vi "GSP_Manager_Wavelength.vi"() -> ()   [LabVIEW 2015]
uses:
  SystemUtil/Command.ctl
  SystemUtil/ScriptArray.ctl
  SystemUtil/Script.ctl
  wavelength_parameters.ctl
  movetypes.ctl
  SystemUtil/MotorStates.ctl
  SystemUtil/ThreadStates.ctl
  Log/LogItem.ctl
  GSP_Wavelength_Global.vi
  GUI/GSP_GUI_global.vi
panel:
  out "Camera":dbl
  out "Grating":dbl
  out "Array":T1(array[cluster])
  in  "Set":bool
  in  "Load Littrow":bool
  in  "Select Mode:":u16(ring) items=["Custom", "Imaging", "300 All", "600 UV", "600 Blue", "600 Mid", "600 Red", "1200 m0", "1200 m1", "1200 m2", "1200 m3", "1200 m4", "1200 m5", "1200 m6", "1200 m7", "1200 RESOLVE", "400 m1", "400 m2", "930 m1", "930 m2", "930 m3", "930 m4", "930 m5", "930 m6", "400WD", "930TP", "400Fermi", "400Padgett", "400Lewis", "400Crotts", "600BLee", "600RLee", "400WW", "ZZ Ceti Red", "ZZ Ceti Blue"]
  in  "Central wavelength(nm)":dbl
  in  "CS Target":dbl caption="Target" format="%.5f"
  out "CS Angle":dbl caption="Actual" format="%.5f"
  in  "GS Target":dbl caption="Target" format="%.5f"
  out "GS Angle":dbl caption="Actual" format="%.5f"
  out "Last Error":errorcluster
  in  "CommandQ":string
  # "Grating"
  # "Camera"
  # "Littrow Configuration"
  # "Wavelength Angles"
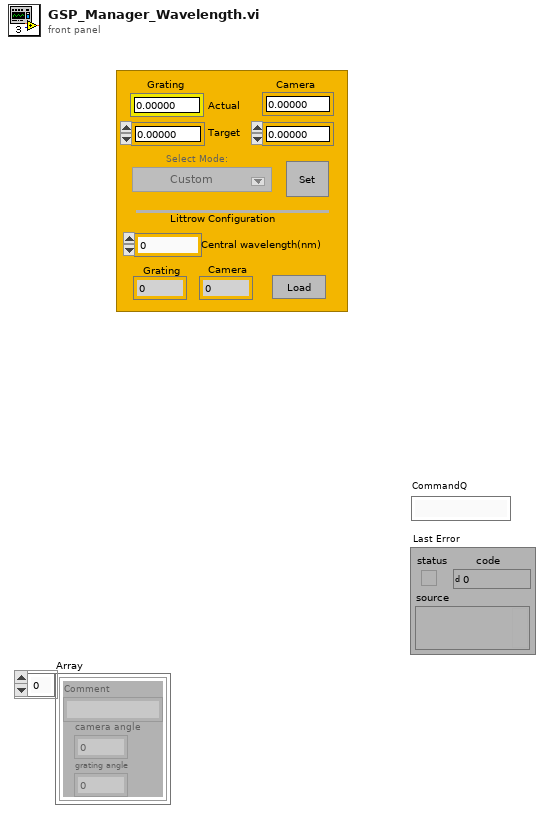
[diagram p1: front panel]
types:
  T1 = cluster{"Comment":string, "camera angle":dbl, "grating angle":dbl}[]
  T2 = typedef "ScriptArray.ctl" = T3[]
  T3 = typedef "Script.ctl" = cluster{"Current Step":i32, "Commands":cluster{"Command":string, "Parameters":string}[]}
  T4 = typedef "Command.ctl" = cluster{"Command":string, "Parameter":string}
  T5 = cluster{"CS - Ext Move Mem Address":i32, "CS - Home Mem Address":i32, "CS - Int Move Mem Address":i32, "GS - Move Mem Address":i32, "GS - Home Mem Address":i32}
  T6 = typedef "wavelength_parameters.ctl" = cluster{"Camera Angle":dbl, "Grating  Angle":dbl, "Move type":T7}
  T7 = typedef "movetypes.ctl" = u16
  T8 = enum16{"POL (0)", "CPL (1)", "HLT (2)", "STP (3)", "RST (4)", "RVN (5)", "RPB (6)", "CLP (8)", "SDL (9)", "RUN (10)", "WRI (11)", "RRG (12)", "SPR (13)", "LPR (14)", "VMI (15)", "SSP (17)", "SSE (18)", "RIS (20)", "RIO (21)", "IMW (25)", "END (128)", "MAV (134)", "MRV (135)", "JRE (137)", "WCL (138)", "WCW (139)", "DLY (140)", "WDL (141)", "GCL (142)", "GOP (143)", "ZTG (144)", "ZTP (145)", "TTP (146)", "CME (147)", "CTC (148)", "TQL (149)", "AHC (150)", "ERL (151)", "OLP (152)", "WRP (154)", "IDT (155)", "LRP (156)", "VMP (159)", "RAV (160)", "RRV (161)", "JMP (162)", "JOI (162)", "CIS (163)", "CKS (164)", "CLC (165)", "KMC (167)", "MCT (168)", "FLC (169)", "EEM (170)", "DDB (171)", "DEM (171)", "PAC (172)", "ADL (173)", "BRT (174)", "MAT (176)", "MRT (177)", "RAT (178)", "RRT (179)", "SSD (180)", "KMR (181)", "KED (182)", "KDD (183)", "DIR (184)", "PRO (185)", "SIF (186)", "EDL (187)", "CIO (188)", "MDS (189)", "MDC (190)", "MDT (191)", "SEE (192)", "ARI (193)", "WBS (194)", "SCF (195)", "RSM (196)", "RLM (197)", "RSN (198)", "RLN (199)", "PCL (201)", "PCI (201)", "PRT (202)", "PRI (202)", "WBE (204)", "SOB (205)", "COB (206)", "ACR (207)", "PLR (208)", "CAI (211)", "LVT (212)", "OVT (213)", "MTT (214)", "CLC (215)", "PIM (216)", "VIM (217)", "TIM (218)", "AHM (219)", "SSL (221)", "TRU (222)", "RSD (223)", "EMT (225)", "DMT (226)", "EMD (227)", "DMD (228)", "HSM (229)", "AHD (230)", "PCM (231)", "PCG (232)", "XRV (233)", "XAV (234)", "XRT (235)", "XAT (236)", "GOC (237)", "JNA (238)", "JOR (239)", "PMC (240)", "PMV (241)", "PMX (242)", "DLC (243)", "SLC (244)", "PCP (245)", "ATR (248)", "PMO (249)", "JAN (250)", "EDH (251)", "DIF (252)", "IMS (253)", "IMQ (254)"}
  T9 = typedef "MotorStates.ctl" = enum16{"Ready", "Moving", "Uninitialized", "Error"}
  T10 = typedef "ThreadStates.ctl" = enum16{"Waiting", "Scripting", "Uninitialized", "Error"}
  T11 = enum16{"Launch", "Log", "Open", "Close", "Shutdown"}
  T12 = typedef "LogItem.ctl" = cluster{"error in (no error)":errorcluster, "Source":string, "Comment ":string}
  T13 = cluster{"Comment":string, "camera angle":dbl, "grating angle":dbl}
  T14 = cluster{"Comment":string, "lines/mm":i32, "modulation":dbl, "thickness (mm)":dbl}
  T15 = cluster{"Mount Az":dbl, "Mount El":dbl, "RA":string, "DEC":string, "Hour Angle":string, "Airmass":dbl, "Focus":dbl, "Rotator Angle":dbl, "Rotator Location":string, "Dome Shutter":string, "Dome Az":dbl, "Date":string, "UT Time":string, "Sidereal Time":string, "Position Angle":dbl, "Seeing":dbl, "OBSRA":string, "OBSDEC":string, "Position ADC":string, "Position ADC 2":string, "Bulb":bool, "Ar":bool, "Cu":bool, "Dome":bool, "Fe":bool, "Hg(Ar)":bool, "Ne":bool, "Quartz":bool, "Dome Percent":dbl, "Quartz Percent":dbl}
  T16 = cluster{"Command":string, "data string":string}[]
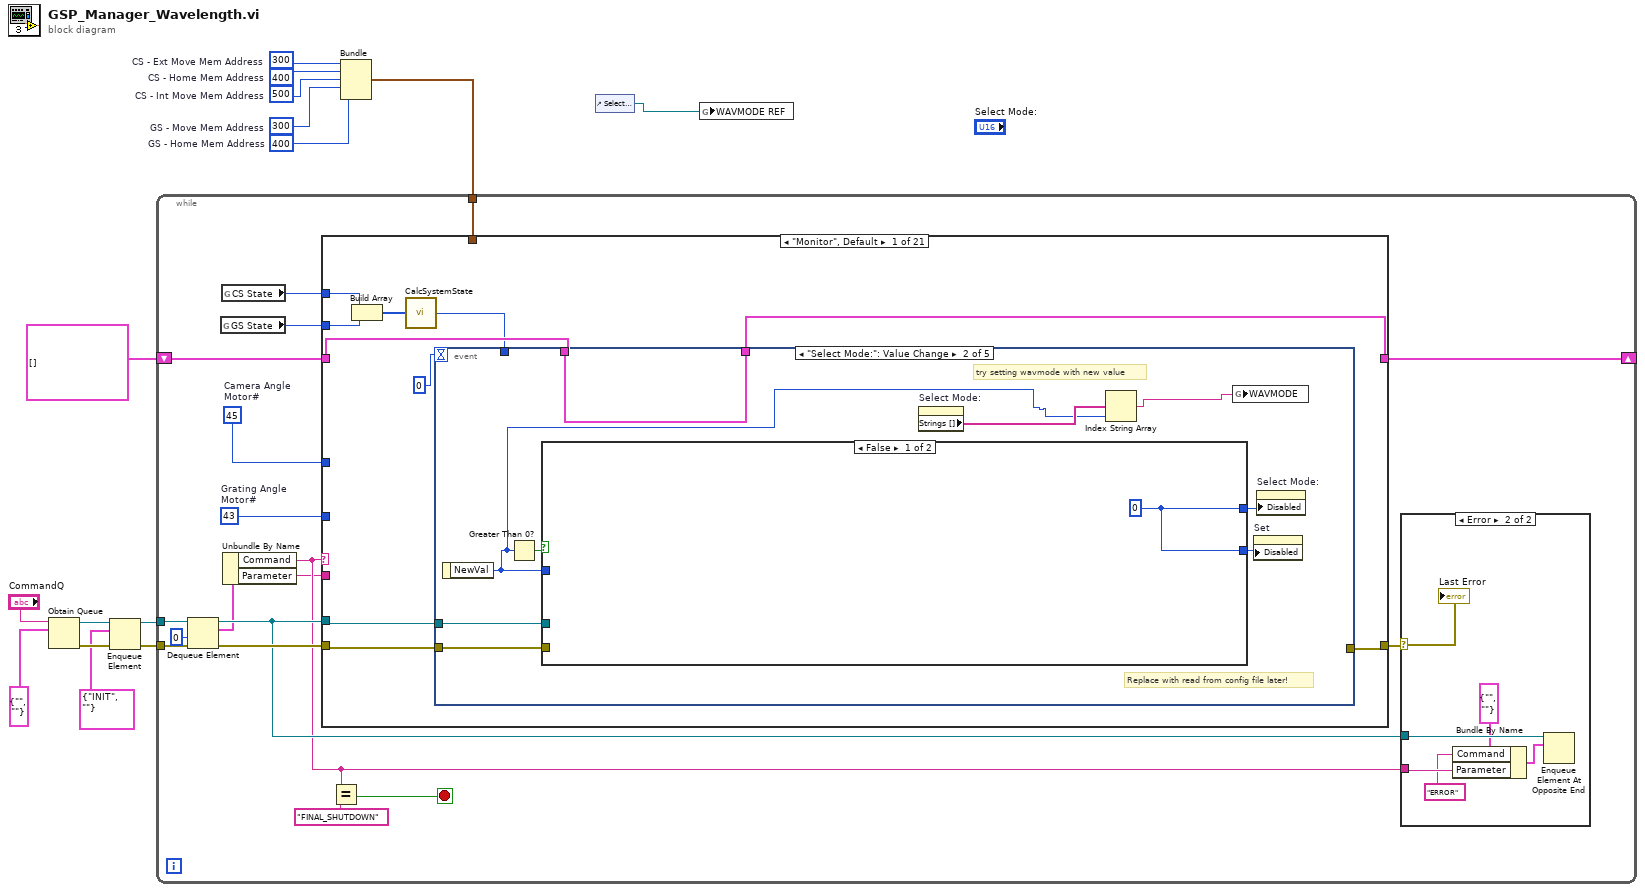
[diagram p0: block diagram]
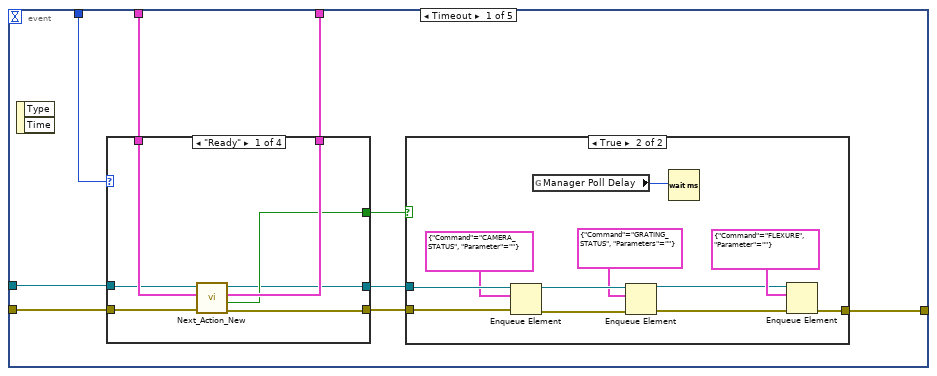
[diagram p3: hidden frame]
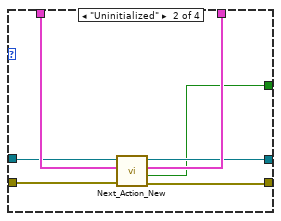
[diagram p5: hidden frame]
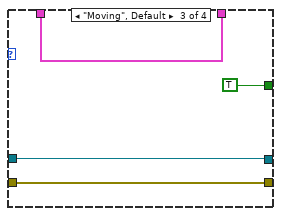
[diagram p6: hidden frame]
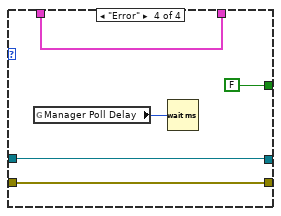
[diagram p7: hidden frame]
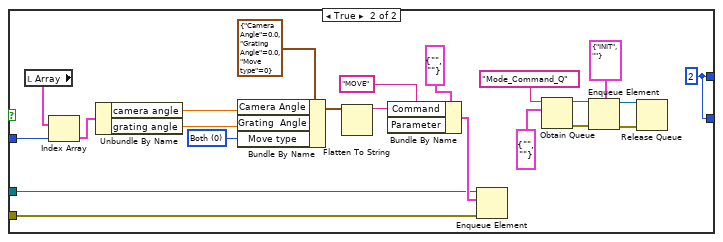
[diagram p8: hidden frame]
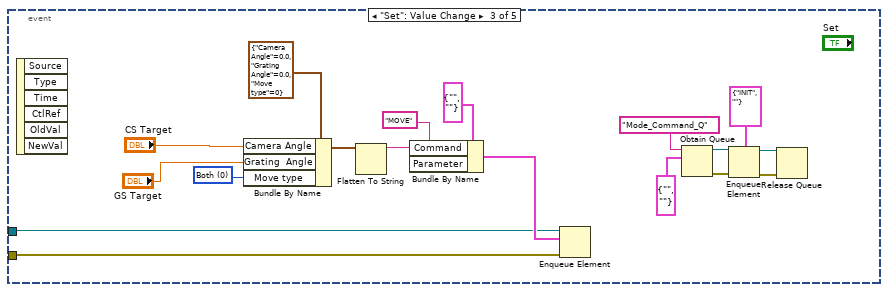
[diagram p9: hidden frame]
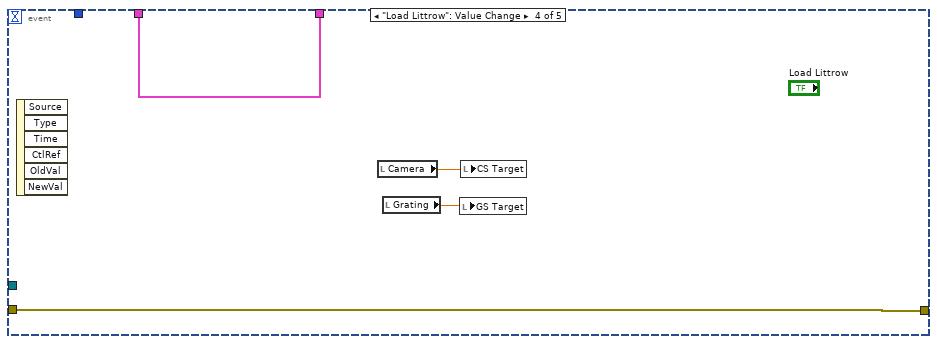
[diagram p10: hidden frame]
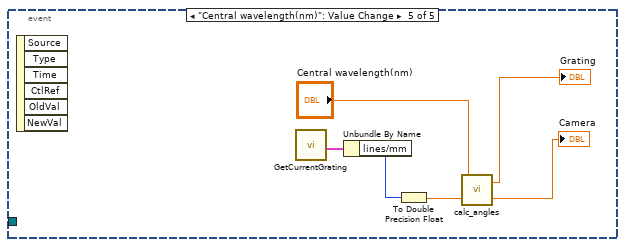
[diagram p11: hidden frame]
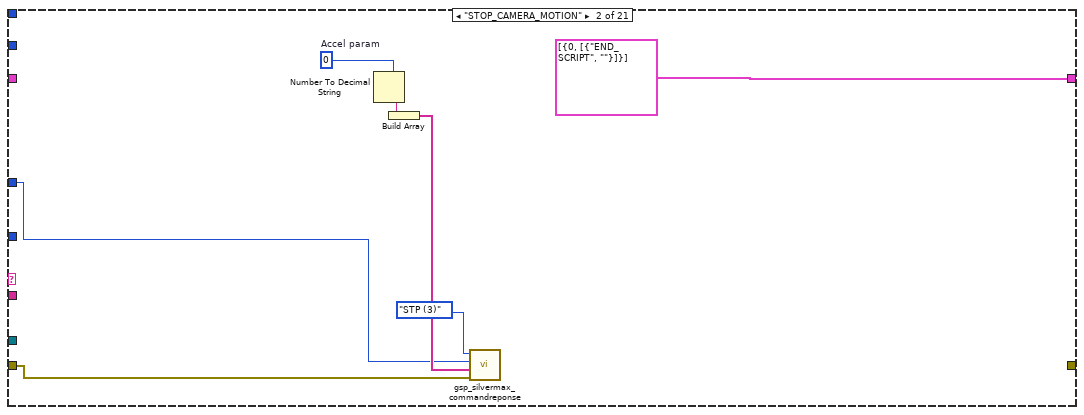
[diagram p12: hidden frame]
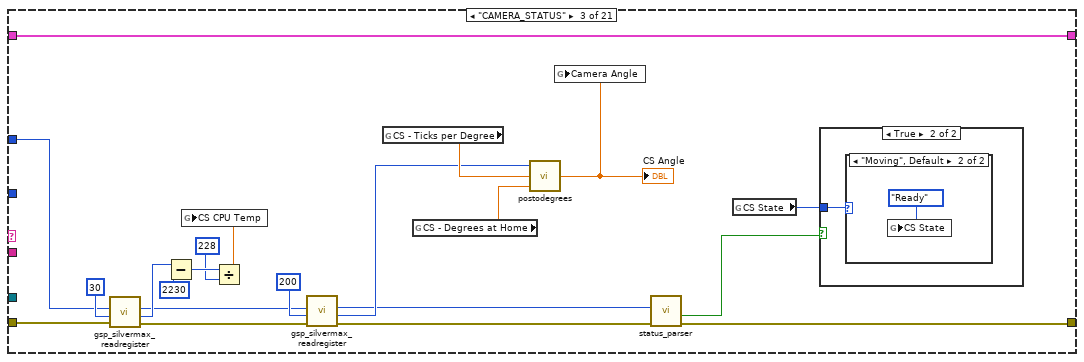
[diagram p13: hidden frame]
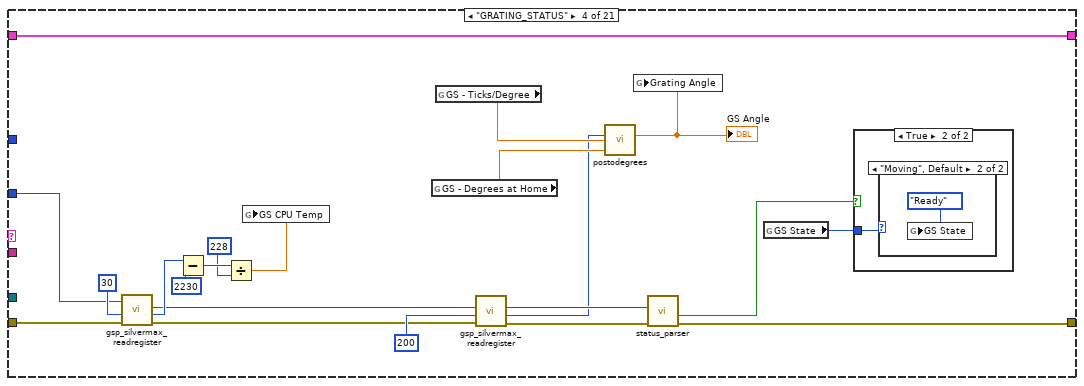
[diagram p16: hidden frame]
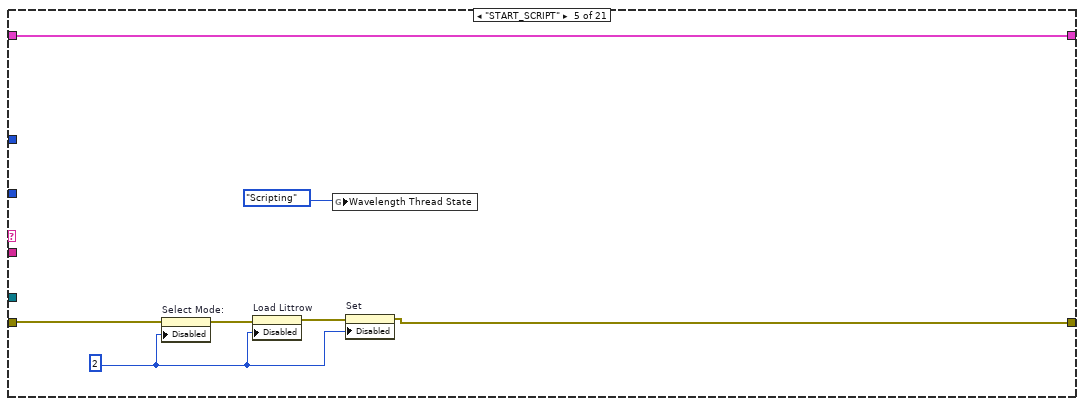
[diagram p19: hidden frame]
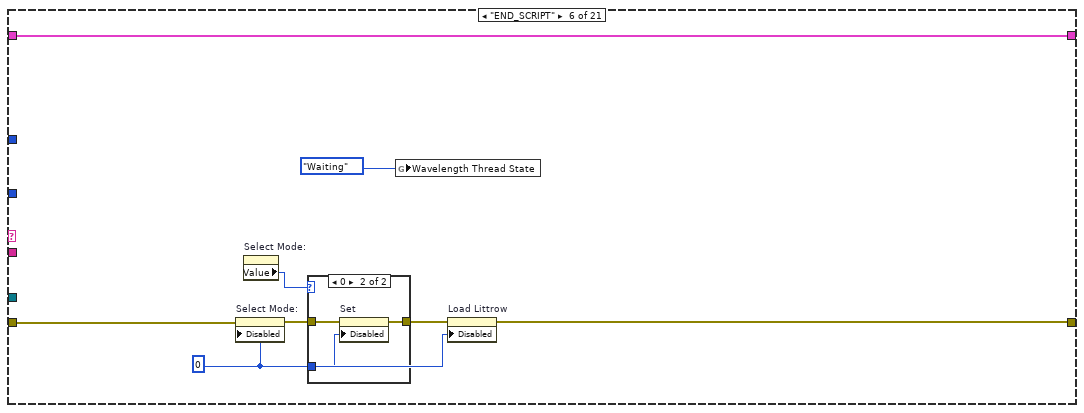
[diagram p20: hidden frame]
diagram:
  w3 = 400  # GS - Home Mem Address
  w6 = 400  # CS - Home Mem Address
  w4 = 300  # GS - Move Mem Address
  w7 = 300  # CS - Ext Move Mem Address
  w5 = 500  # CS - Int Move Mem Address
  n1 = Obtain Queue(name (unnamed)="CommandQ", element data type=T4 {"Command"="", "Parameter"=""} ("Command")) -> (queue out=w13:refnum<queue>, error out=w12:errorcluster)  [unwired: 3 in, 1 out]
  n2 = Enqueue Element(queue=w13, element=T4 {"Command"="INIT", "Parameter"=""}, error in (no error)=w12) -> (queue out=w14:refnum<queue>, error out=w11:errorcluster)  [unwired: 1 in, 1 out]
  n3 = Bundle("CS - Ext Move Mem Address"=w7, "CS - Home Mem Address"=w6, "CS - Int Move Mem Address"=w5, "GS - Move Mem Address"=w4, "GS - Home Mem Address"=w3) -> (w2:T5)  [unwired: 1 in]
  n4 = while {
    tunnel: w14 -> [w33]
    tunnel: w11 -> [w32]
    shift-right: [w25] -> _
    shift-left: T2 [] ("Operations") -> [w27]
    tunnel: w2 -> [w16]
    stop <- w22 stop-if-true
    w21 = u8 43  # Grating Angle Motor#
    w20 = u8 45  # Camera Angle Motor#
    n5 = Dequeue Element(queue=w33, timeout in ms (-1)=0, error in (no error)=w32) -> (queue out=w29:refnum<queue>, element=w24:T4, error out=w31:errorcluster)  [unwired: 1 out]
    n6 = global read "GSP_Wavelength_Global.vi" "GS State"() -> (w17:T9)
    n7 = global read "GSP_Wavelength_Global.vi" "CS State"() -> (w18:T9)
    n8 = Unbundle By Name(w24) -> ("Command"=w23:string, "Parameter"=w19:string)
    n9 = case shown="\"Monitor\", Default" w23 {
      tunnel: w31 -> [w45 w155 w166 w196 w211 w219 w229 w249 w292 w296 w314 _ w362 w384 w406 w429 w469 w515 w522 w523 _]
      tunnel: w29 -> [w46 _ _ _ _ _ _ _ _ _ _ _ _ _ _ _ w471 w514 _ _ w552]
      tunnel: [w49 _ w163 w186 w208 w215 w231 w248 w292 w296 w314 w354 w374 w396 w418 w434 w470 w510 w522 w537 _] -> w30
      tunnel: w27 -> [w48 _ w181 w204 w213 w221 w238 w252 w293 w302 w316 w341 w371 w393 w415 w435 w472 w513 w521 w534 w545]
      tunnel: [w47 T2 [{"Current Step"=0, "Commands"=[{"Command"="END_SCRIPT", "Parameters"=""}]}] ("Operations") w181 w204 w213 w221 w238 w250 w293 w301 w315 w341 w371 w393 w415 w435 w468 w513 w520 w534 w544] -> w25
      tunnel: w19 -> [_ _ _ _ _ _ _ w251 _ _ _ w348 w369 w391 w414 w452 _ _ _ _ _]
      tunnel: w21 -> [_ _ _ w197 _ _ _ _ _ _ _ _ _ _ w409 w438 _ _ _ w527 _]
      tunnel: w20 -> [_ w156 w167 _ _ _ _ _ _ _ _ w344 w370 w392 _ w449 _ _ _ w528 _]
      tunnel: w18 -> [w44 _ _ _ _ _ _ w246 _ _ w311 _ _ _ _ _ _ _ _ _ _]
      tunnel: w17 -> [w43 _ _ _ _ _ _ w245 _ _ w310 _ _ _ _ _ _ _ _ _ _]
      tunnel: w16 -> [_ _ _ _ _ _ _ _ _ _ _ w343 w364 w386 w408 w448 _ _ _ w526 _]
      frame "Monitor", Default {
        n10 = Build Array(w44, w43) -> (w42:T9[])
        n11 = call "CalcSystemState.vi"("Motor States"=w42) -> ("system state"=w41:T9)
        n12 = event shown="[1] \"Select Mode:\": Value Change" {
          selector: _ -> [_ _ _ _ _]
          dyn-events: _ -> [_ _ _ _ _]
          timeout: 0 -> [_ _ _ _ _]
          tunnel: [w55 _ _ w147 _] -> w49
          tunnel: w48 -> [w54 w100 _ w146 _]
          tunnel: [w53 w100 _ w146 _] -> w47
          tunnel: w46 -> [w52 w102 w137 _ _]
          tunnel: w45 -> [w51 w101 w136 w147 _]
          tunnel: w41 -> [w50 _ _ _ _]
          event Timeout {
            n13 = event-data() -> ()  [unwired: 1 in, 2 out]
            n14 = case shown="\"Ready\"" w50 {
              tunnel: w52 -> [w73 w80 w87 w90]
              tunnel: w51 -> [w77 w84 w86 w92]
              tunnel: [w75 w82 w86 w92] -> w58
              tunnel: w54 -> [w76 w83 w88 w93]
              tunnel: [w74 w81 w88 w93] -> w53
              tunnel: [w72 w78 TRUE FALSE] -> w57
              tunnel: [w71 w79 w87 w90] -> w56
              frame "Ready" {
                n15 = call "Next_Action_New.vi"("error in (no error)"=w77, "Operations"=w76, "queue in"=w73) -> ("error out"=w75:errorcluster, "No command?"=w72:bool, "Operations Out"=w74:T2, "queue out"=w71:refnum<queue>)  [unwired: 1 in]
              }
              frame "Uninitialized" {
                n16 = call "Next_Action_New.vi"("error in (no error)"=w84, "Operations"=w83, "queue in"=w80) -> ("error out"=w82:errorcluster, "No command?"=w78:bool, "Operations Out"=w81:T2, "queue out"=w79:refnum<queue>)  [unwired: 1 in]
              }
              frame "Moving", Default {
              }
              frame "Error" {
                n17 = global read "GSP_GUI_global.vi" "Manager Poll Delay"() -> (w91:u32)
                n18 = Wait (ms)(milliseconds to wait=w91) -> ()  [unwired: 1 out]
              }
            }
            n19 = case shown="True" w57 {
              tunnel: w58 -> [w59 w70]
              tunnel: w56 -> [_ w69]
              tunnel: [w59 w60] -> w55
              frame False {
              }
              frame True {
                n20 = Enqueue Element(queue=w69, element=T4 {"Command"="CAMERA_STATUS", "Parameter"=""}, error in (no error)=w70) -> (queue out=w67:refnum<queue>, error out=w66:errorcluster)  [unwired: 1 in, 1 out]
                n21 = global read "GSP_GUI_global.vi" "Manager Poll Delay"() -> (w68:u32)
                n22 = Enqueue Element(queue=w67, element=cluster{"Command":string, "Parameters":string} {"Command"="GRATING_STATUS", "Parameters"=""} ("Default Command"), error in (no error)=w66) -> (queue out=w62:refnum<queue>, error out=w61:errorcluster)  [unwired: 1 in, 1 out]
                n23 = Wait (ms)(milliseconds to wait=w68) -> ()  [unwired: 1 out]
                n24 = Enqueue Element(queue=w62, element=T4 {"Command"="FLEXURE", "Parameter"=""}, error in (no error)=w61) -> (error out=w60:errorcluster)  [unwired: 1 in, 2 out]
              }
            }
          }
          event "Select Mode:": Value Change {
            # "try setting wavmode with new value"
            # "Replace with read from config file later!"
            n25 = event-data() -> ("NewVal"=w94:u16)  [unwired: 1 in]
            n26 = Greater Than 0?(x=w94) -> (x > 0?=w99:bool)
            n27 = case shown="False" w99 {
              tunnel: w94 -> [_ w115]
              tunnel: w102 -> [_ w118]
              tunnel: w101 -> [_ w117]
              tunnel: [w103 w116] -> w98
              tunnel: [w103 w116] -> w97
              frame False {
                w103 = u8 0 ("Disabled")
              }
              frame True {
                w116 = u8 2 ("Disabled")
                w119 = T7 0 items=["Both", "Grating Only", "Camera Only"] ("Move type")
                n28 = local read "Array"() -> (w114:T1)
                n29 = Index Array(array=w114, index=w115) -> (element=w113:T13)
                n30 = Unbundle By Name(w113) -> ("camera angle"=w112:dbl, "grating angle"=w111:dbl)
                n31 = Bundle By Name(cluster=T6 {"Camera Angle"=0.0, "Grating  Angle"=0.0, "Move type"=0} ("Wavelength Parameters"), "Camera Angle"=w112, "Grating  Angle"=w111, "Move type"=w119) -> (w120:T6)
                n32 = Flatten To String(anything=w120) -> (data string=w123:string)  [unwired: 3 in, 2 out]
                n33 = Bundle By Name(cluster=T4 {"Command"="", "Parameter"=""} ("element"), "Command"="MOVE", "Parameter"=w123) -> (w124:T4)
                n34 = Enqueue Element(queue=w118, element=w124, error in (no error)=w117) -> ()  [unwired: 1 in, 3 out]
                n35 = Obtain Queue(name (unnamed)="Mode_Command_Q", element data type=T4 {"Command"="", "Parameter"=""} ("element")) -> (queue out=w110:refnum<queue>, error out=w109:errorcluster)  [unwired: 3 in, 1 out]
                n36 = Enqueue Element(queue=w110, element=T4 {"Command"="INIT", "Parameter"=""}, error in (no error)=w109) -> (queue out=w105:refnum<queue>, error out=w104:errorcluster)  [unwired: 1 in, 1 out]
                n37 = Release Queue(queue=w105, error in (no error)=w104) -> ()  [unwired: 1 in, 3 out]
              }
            }
            n38 = property on="Select Mode:" class="Ring (strict)"() -> ("Strings []"=w96:string[])  [unwired: 2 in, 2 out]
            n39 = Index String Array(1:w94, 2:w96) -> (0:w95:string)  [unwired: 1 in]
            n40 = global write "GSP_Wavelength_Global.vi" "WAVMODE"(w95) -> ()
            n41 = property on="Set" class="Bool"("Disabled"=w97) -> ()  [unwired: 2 in, 2 out]
            n42 = property on="Select Mode:" class="Ring (strict)"("Disabled"=w98) -> ()  [unwired: 2 in, 2 out]
          }
          event "Set": Value Change {
            w138 = T7 0 items=["Both", "Grating Only", "Camera Only"] ("Move type")
            n43 = event-data() -> ()  [unwired: 1 in, 6 out]
            n44 = Bundle By Name(cluster=T6 {"Camera Angle"=0.0, "Grating  Angle"=0.0, "Move type"=0} ("Wavelength Parameters"), "Camera Angle"="CS Target", "Grating  Angle"="GS Target", "Move type"=w138) -> (w139:T6)
            n45 = Flatten To String(anything=w139) -> (data string=w141:string)  [unwired: 3 in, 2 out]
            n46 = Bundle By Name(cluster=T4 {"Command"="", "Parameter"=""} ("element"), "Command"="MOVE", "Parameter"=w141) -> (w142:T4)
            n47 = Enqueue Element(queue=w137, element=w142, error in (no error)=w136) -> ()  [unwired: 1 in, 3 out]
            n48 = Obtain Queue(name (unnamed)="Mode_Command_Q", element data type=T4 {"Command"="", "Parameter"=""} ("element")) -> (queue out=w132:refnum<queue>, error out=w131:errorcluster)  [unwired: 3 in, 1 out]
            n49 = Enqueue Element(queue=w132, element=T4 {"Command"="INIT", "Parameter"=""}, error in (no error)=w131) -> (queue out=w127:refnum<queue>, error out=w126:errorcluster)  [unwired: 1 in, 1 out]
            n50 = Release Queue(queue=w127, error in (no error)=w126) -> ()  [unwired: 1 in, 3 out]
          }
          event "Load Littrow": Value Change {
            n51 = event-data() -> ()  [unwired: 1 in, 6 out]
            n52 = local read "Camera"() -> (w145:dbl)
            n53 = local read "Grating"() -> (w144:dbl)
            n54 = local write "GS Target"(w144) -> ()
            n55 = local write "CS Target"(w145) -> ()
          }
          event "Central wavelength(nm)": Value Change {
            n56 = event-data() -> ()  [unwired: 1 in, 6 out]
            n57 = call "GetCurrentGrating.vi"() -> ("Current Grating"=w153:T14)
            n58 = Unbundle By Name(w153) -> ("lines/mm"=w151:i32)
            n59 = To Double Precision Float(number=w151) -> (double precision float=w152:dbl)
            n60 = call "calc_angles.vi"("lines/mm"=w152, "Central Wavlength (nm)"="Central wavelength(nm)") -> ("camera angle"=→"Camera":dbl, "grating angle"=→"Grating":dbl)
          }
        }
      }
      frame "STOP_CAMERA_MOTION" {
        w159 = u8 0  # Accel param
        n61 = Number To Decimal String(number=w159) -> (decimal integer string=w160:string)  [unwired: 1 in]
        n62 = Build Array(w160) -> (w157:string[])
        n63 = call "gsp_silvermax_commandreponse.vi"("error in (no error)"=w155, "Parameters (none)"=w157, "Motor #"=w156, "Command"=T8."STP (3)") -> ()  [unwired: 4 out]
      }
      frame "CAMERA_STATUS" {
        n64 = call "gsp_silvermax_readregister.vi"("error in (no error)"=w166, "Register# (0)"=u8 30, "Motor #"=w167) -> ("error out"=w165:errorcluster, "Register Value"=w172:i32, "Motor # dup"=w164:u8)  [unwired: 2 in, 2 out]
        n65 = Subtract(x=w172, y=2230) -> (x-y=w171:i32)
        n66 = Divide(x=w171, y=228) -> (x/y=w169:dbl)
        n67 = global write "GSP_Wavelength_Global.vi" "CS CPU Temp"(w169) -> ()
        n68 = call "gsp_silvermax_readregister.vi"("error in (no error)"=w165, "Register# (0)"=u8 200, "Motor #"=w164) -> ("error out"=w179:errorcluster, "Register Value"=w176:i32, "Motor # dup"=w174:u8)  [unwired: 2 in, 2 out]
        n69 = global read "GSP_Wavelength_Global.vi" "CS - Ticks per Degree"() -> (w178:dbl)
        n70 = global read "GSP_Wavelength_Global.vi" "CS - Degrees at Home"() -> (w177:dbl)
        n71 = call "postodegrees.vi"("Degrees @ Home (15.00)"=w177, "Ticks per degree (28571.43)"=w178, "Ext Position"=w176) -> ("Degrees"=w161:dbl)  [unwired: 2 in]
        "CS Angle" <- w161
        n72 = global write "GSP_Wavelength_Global.vi" "Camera Angle"(w161) -> ()
        n73 = call "status_parser.vi"("error in (no error)"=w179, "Motor #"=w174) -> ("error out"=w163:errorcluster, "Program Complete?"=w180:bool)  [unwired: 3 in, 1 out]
        n74 = global read "GSP_Wavelength_Global.vi" "CS State"() -> (w162:T9)
        n75 = case shown="True" w180 {
          tunnel: w162 -> [_ w182]
          frame False {
          }
          frame True {
            n76 = case shown="\"Moving\", Default" w182 {
              frame "Uninitialized" {
              }
              frame "Moving", Default {
                n77 = global write "GSP_Wavelength_Global.vi" "CS State"(MotorStates."Ready" ("Mode")) -> ()
              }
            }
          }
        }
      }
      frame "GRATING_STATUS" {
        n78 = call "gsp_silvermax_readregister.vi"("error in (no error)"=w196, "Register# (0)"=u8 30, "Motor #"=w197) -> ("error out"=w188:errorcluster, "Register Value"=w202:i32, "Motor # dup"=w187:u8)  [unwired: 2 in, 2 out]
        n79 = Subtract(x=w202, y=2230) -> (x-y=w201:i32)
        n80 = Divide(x=w201, y=228) -> (x/y=w199:dbl)
        n81 = global write "GSP_Wavelength_Global.vi" "GS CPU Temp"(w199) -> ()
        n82 = global read "GSP_Wavelength_Global.vi" "GS - Degrees at Home"() -> (w191:dbl)
        n83 = global read "GSP_Wavelength_Global.vi" "GS - Ticks/Degree"() -> (w192:dbl)
        n84 = call "gsp_silvermax_readregister.vi"("error in (no error)"=w188, "Register# (0)"=u8 200, "Motor #"=w187) -> ("error out"=w195:errorcluster, "Register Value"=w190:i32, "Motor # dup"=w194:u8)  [unwired: 2 in, 2 out]
        n85 = call "postodegrees.vi"("Degrees @ Home (15.00)"=w191, "Ticks per degree (28571.43)"=w192, "Ext Position"=w190) -> ("Degrees"=w184:dbl)  [unwired: 2 in]
        "GS Angle" <- w184
        n86 = global write "GSP_Wavelength_Global.vi" "Grating Angle"(w184) -> ()
        n87 = call "status_parser.vi"("error in (no error)"=w195, "Motor #"=w194) -> ("error out"=w186:errorcluster, "Program Complete?"=w193:bool)  [unwired: 3 in, 1 out]
        n88 = global read "GSP_Wavelength_Global.vi" "GS State"() -> (w185:T9)
        n89 = case shown="True" w193 {
          tunnel: w185 -> [_ w205]
          frame False {
          }
          frame True {
            n90 = case shown="\"Moving\", Default" w205 {
              frame "Uninitialized" {
              }
              frame "Moving", Default {
                n91 = global write "GSP_Wavelength_Global.vi" "GS State"(MotorStates."Ready" ("Grating Mode")) -> ()
              }
            }
          }
        }
      }
      frame "START_SCRIPT" {
        w207 = u8 2 ("Disabled")
        n92 = property on="Select Mode:" class="Ring (strict)"(error in=w211, "Disabled"=w207) -> (error out=w210:errorcluster)  [unwired: 1 in, 1 out]
        n93 = property on="Load Littrow" class="Bool"(error in=w210, "Disabled"=w207) -> (error out=w209:errorcluster)  [unwired: 1 in, 1 out]
        n94 = global write "GSP_Wavelength_Global.vi" "Wavelength Thread State"(ThreadStates."Scripting" ("Thread state")) -> ()
        n95 = property on="Set" class="Bool"(error in=w209, "Disabled"=w207) -> (error out=w208:errorcluster)  [unwired: 1 in, 1 out]
      }
      frame "END_SCRIPT" {
        w218 = u8 0 ("Disabled")
        n96 = property on="Select Mode:" class="Ring (strict)"(error in=w219, "Disabled"=w218) -> (error out=w217:errorcluster)  [unwired: 1 in, 1 out]
        n97 = property on="Select Mode:" class="Ring (strict)"() -> ("Value"=w214:u16)  [unwired: 2 in, 2 out]
        n98 = case shown="0" w214 {
          tunnel: w218 -> [_ w225]
          tunnel: w217 -> [w222 w224]
          tunnel: [w222 w223] -> w216
          frame 1, Default {
          }
          frame 0 {
            n99 = property on="Set" class="Bool"(error in=w224, "Disabled"=w225) -> (error out=w223:errorcluster)  [unwired: 1 in, 1 out]
          }
        }
        n100 = global write "GSP_Wavelength_Global.vi" "Wavelength Thread State"(ThreadStates."Waiting" ("Thread state")) -> ()
        n101 = property on="Load Littrow" class="Bool"(error in=w216, "Disabled"=w218) -> (error out=w215:errorcluster)  [unwired: 1 in, 1 out]
      }
      frame "INIT" {
        w232 = u8 2 ("Disabled")
        w237 = MotorStates."Uninitialized" ("Camera Mode")
        n102 = global read "GSP_GUI_global.vi" "Standard Observing Mode Names"() -> (w227:string[])
        n103 = global read "GSP_GUI_global.vi" "Standard Observing Modes File"() -> (w230:path)
        n104 = for {
          tunnel: w227 -> [w243] mode=indexing
          tunnel: w230 -> [w244]
          tunnel: w229 -> [w242]
          tunnel: [w241] -> w228
          tunnel: [w240] -> w226 mode=indexing
          n105 = call "get_std_observing_modes.vi"("error in (no error)"=w242, "mode name"=w243, "configuration file path"=w244) -> ("error out"=w241:errorcluster, "Standard Mode Info"=w240:T13)  [unwired: 3 in]
        }
        "Array" <- w226
        n106 = property on="Select Mode:" class="Ring (strict)"(error in=w228, "Disabled"=w232) -> (error out=w234:errorcluster)  [unwired: 1 in, 1 out]
        n107 = property on="Select Mode:" class="Ring (strict)"("Strings []"=w227) -> ()  [unwired: 2 in, 2 out]
        n108 = property on="Set" class="Bool"(error in=w234, "Disabled"=w232) -> (error out=w233:errorcluster)  [unwired: 1 in, 1 out]
        n109 = property on="Load Littrow" class="Bool"(error in=w233, "Disabled"=w232) -> (error out=w231:errorcluster)  [unwired: 1 in, 1 out]
        n110 = global write "GSP_Wavelength_Global.vi" "Flexure Active"(FALSE ("Flexure Active")) -> ()
        n111 = global write "GSP_Wavelength_Global.vi" "WL Online"(TRUE ("CS Online")) -> ()
        n112 = global write "GSP_Wavelength_Global.vi" "Wavelength Thread State"(ThreadStates."Uninitialized" ("Thread state")) -> ()
        n113 = global write "GSP_Wavelength_Global.vi" "CS State"(w237) -> ()
        n114 = global write "GSP_Wavelength_Global.vi" "GS State"(w237) -> ()
      }
      frame "MOVE" {
        n115 = call "Slit_allow_move.vi"("Translation Mode"=w246, "Rotation Mode"=w245) -> ("Allow Move?"=w247:bool)
        n116 = case shown="True" w247 {
          tunnel: w252 -> [w269 w284]
          tunnel: w251 -> [w267 _]
          tunnel: [w268 w284] -> w250
          tunnel: w249 -> [w256 w289]
          tunnel: [w257 w288] -> w248
          frame True {
            n117 = Unflatten From String(type=T6 {"Camera Angle"=0.0, "Grating  Angle"=0.0, "Move type"=0} ("Wavelength Parameters"), binary string=w267) -> (value=w265:T6)  [unwired: 3 in, 2 out]
            n118 = global read "GSP_Wavelength_Global.vi" "Grating Angle"() -> (w255:dbl)
            n119 = global read "GSP_Wavelength_Global.vi" "Camera Angle"() -> (w254:dbl)
            n120 = Unbundle By Name(w265) -> ("Move type"=w253:T7, "Grating  Angle"=w259:dbl, "Camera Angle"=w258:dbl)
            n121 = call "GSP_Wavelength_GenerateScript.vi"("Current Grating"=w255, "Current Camera"=w254, "Target Grating"=w259, "Target Camera"=w258, "Move type"=w253) -> ("Script"=w263:cluster{string, string}[], "AllowMove?"=w264:bool)
            n122 = Build Array (concatenate)(cluster{string, string} {"START_SCRIPT", ""}, w263, cluster{string, string} {"END_SCRIPT", ""}) -> (w261:cluster{string, string}[])
            n123 = case shown="True" w264 {
              tunnel: w269 -> [w276 w281]
              tunnel: [w276 w279] -> w268
              tunnel: w261 -> [_ w278]
              tunnel: w259 -> [_ _]
              tunnel: w258 -> [_ _]
              tunnel: [w271 w277] -> w257
              tunnel: w256 -> [w272 w277]
              frame False {
                w274 = T12 {"error in (no error)"={"status"=FALSE, "code"=0, "source"=""}, "Source"="", "Comment "=""} ("Log")
                n124 = Bundle By Name(cluster=w274, "Comment"="Move request out of bounds", "Source"="Wavlength Manager") -> ()  [unwired: 1 out]
                n125 = call "GSP_Logger_Handler.vi"("error in (no error)"=w272, "Log"=w274, "Actions"=T11."Log") -> ("error out"=w271:errorcluster)  [unwired: 4 in]
              }
              frame True {
                n126 = call "Build_Script.vi"("Commands"=w278) -> ("script out"=w280:T3)  [unwired: 4 in]
                n127 = Insert Into Array(array=w281, new element=w280) -> (w279:T2)  [unwired: 1 in]
              }
            }
          }
          frame False {
            n128 = Bundle By Name(cluster=T12 {"error in (no error)"={"status"=FALSE, "code"=0, "source"=""}, "Source"="", "Comment "=""} ("Log"), "Source"="Wavelength Manager", "Comment"="Cannot perform move") -> (w285:T12)
            n129 = call "GSP_Logger_Handler.vi"("error in (no error)"=w289, "Log"=w285, "Actions"=T11."Log") -> ("error out"=w288:errorcluster)  [unwired: 4 in]
          }
        }
      }
      frame "FLEXURE_ON" {
        n130 = global read "GSP_Wavelength_Global.vi" "Camera Target"() -> (w290:dbl)
        n131 = global write "GSP_Wavelength_Global.vi" "Flexure Active"(TRUE) -> ()
        n132 = global write "GSP_Wavelength_Global.vi" "Camera Flex Target"(w290) -> ()
      }
      frame "FLEXURE_OFF" {
        n133 = global read "GSP_Wavelength_Global.vi" "Camera Target"() -> (w295:dbl)
        n134 = Flatten To String(anything=w295) -> (data string=w294:string)  [unwired: 3 in, 2 out]
        n135 = global write "GSP_Wavelength_Global.vi" "Flexure Active"(FALSE) -> ()
        n136 = Bundle By Name(cluster=T4 {"Command"="", "Parameter"=""} ("element"), "Command"="CAMERA_EXT_MOVE_START", "Parameter"=w294) -> (w297:T4)
        n137 = Build Array(cluster{string, string} {"START_SCRIPT", ""}, w297, cluster{string, string} {"END_SCRIPT", ""}) -> (w299:T4[])
        n138 = call "Build_Script.vi"("Commands"=w299) -> ("script out"=w303:T3)  [unwired: 4 in]
        n139 = Insert Into Array(array=w302, new element=w303) -> (w301:T2)  [unwired: 1 in]
      }
      frame "FLEXURE" {
        n140 = Build Array(w311, w310) -> (w312:T9[])
        n141 = global read "GSP_Wavelength_Global.vi" "Flexure Active"() -> (w313:bool)
        n142 = call "CalcSystemState.vi"("Motor States"=w312) -> ("system state"=w309:T9)
        n143 = Equal?(x=w309, y=MotorStates."Ready") -> (x = y?=w307:bool)
        n144 = And(x=w307, y=w313) -> (x .and. y?=w317:bool)
        n145 = case shown="True" w317 {
          tunnel: w316 -> [w318 w328]
          tunnel: [w318 w327] -> w315
          frame False {
          }
          frame True {
            n146 = call "GetTCSInfo.vi"() -> ("TCSInfo"=w320:T15)
            n147 = global read "GSP_Wavelength_Global.vi" "Camera Flex Target"() -> (w322:dbl)
            n148 = global read "GSP_Wavelength_Global.vi" "Camera Target"() -> (w329:dbl)
            n149 = global read "GSP_Wavelength_Global.vi" "B1"() -> (w330:dbl)
            n150 = Unbundle By Name(w320) -> ("Rotator Angle"=w319:dbl)
            n151 = call "CalcCameraFlex.vi"("Camera Target"=w329, "B1"=w330, "Rotator Position"=w319) -> ("Camera Flex Target"=w325:dbl)  [unwired: 1 out]
            n152 = global read "GSP_Wavelength_Global.vi" "Flex_Max"() -> (w326:dbl)
            n153 = Subtract(x=w325, y=w322) -> (x-y=w324:dbl)
            n154 = Absolute Value(x=w324) -> (abs(x)=w323:dbl)
            n155 = Greater?(x=w323, y=w326) -> (0:w321:bool)
            n156 = case shown="True" w321 {
              tunnel: w328 -> [w331 w333]
              tunnel: w325 -> [_ w334]
              tunnel: [w331 w335] -> w327
              frame False {
              }
              frame True {
                n157 = Flatten To String(anything=w334) -> (data string=w336:string)  [unwired: 3 in, 2 out]
                n158 = Bundle("Command"="CAMERA_FLEX_MOVE_START", "data string"=w336) -> (w337:cluster{"Command":string, "data string":string})  [unwired: 1 in]
                n159 = Build Array(w337) -> (w332:T16)
                n160 = call "Build_Script.vi"("Commands"=w332) -> ("script out"=w338:T3)  [unwired: 4 in]
                n161 = Insert Into Array(array=w333, new element=w338) -> (w335:T2)  [unwired: 1 in]
              }
            }
          }
        }
      }
      frame "CAMERA_INT_MOVE_START" {
        w347 = 0.0  # Degrees
        n162 = Unflatten From String(type=w347, binary string=w348) -> (value=w340:dbl)  [unwired: 3 in, 2 out]
        n163 = Unbundle By Name(w343) -> ("CS - Int Move Mem Address"=w342:i32)
        n164 = global write "GSP_Wavelength_Global.vi" "Camera Target"(w340) -> ()
        n165 = local write "CS Target"(w340) -> ()
        n166 = global read "GSP_Wavelength_Global.vi" "CS - Degrees at Home"() -> (w346:dbl)
        n167 = call "degreestopos.vi"("Degrees @ Home (15.00)"=w346, "Ticks per degree (28571.43)"=1960.0, "Degrees"=w340) -> ("Position"=w351:i32)  [unwired: 2 in]
        n168 = Number To Decimal String(number=w342) -> (decimal integer string=w353:string)  [unwired: 1 in]
        n169 = call "gsp_silvermax_writeregister.vi"("Register Value"=w351, "Motor #"=w344, "Register# (0)"=u8 25) -> ("error out"=w356:errorcluster, "Motor # dup"=w355:u8)  [unwired: 3 in]
        n170 = Build Array(w353) -> (w352:string[])
        n171 = call "gsp_silvermax_commandreponse.vi"("error in (no error)"=w356, "Parameters (none)"=w352, "Motor #"=w355, "Command"=T8."LRP (156)") -> ("error out"=w349:errorcluster)  [unwired: 3 out]
        n172 = case shown="No Error" w349 {
          selector: w349 -> [w359 w360]
          tunnel: [w359 w360] -> w354
          frame No Error {
            n173 = global write "GSP_Wavelength_Global.vi" "CS State"(MotorStates."Moving" ("Mode")) -> ()
          }
          frame Error {
          }
        }
      }
      frame "CAMERA_EXT_MOVE_START" {
        w368 = 0.0  # Degrees
        n174 = Unflatten From String(type=w368, binary string=w369) -> (value=w361:dbl)  [unwired: 3 in, 2 out]
        n175 = global write "GSP_Wavelength_Global.vi" "Camera Target"(w361) -> ()
        n176 = Unbundle By Name(w364) -> ("CS - Ext Move Mem Address"=w363:i32)
        n177 = local write "CS Target"(w361) -> ()
        n178 = global read "GSP_Wavelength_Global.vi" "CS - Degrees at Home"() -> (w366:dbl)
        n179 = global read "GSP_Wavelength_Global.vi" "CS - Ticks per Degree"() -> (w367:dbl)
        n180 = call "degreestopos.vi"("Degrees @ Home (15.00)"=w366, "Ticks per degree (28571.43)"=w367, "Degrees"=w361) -> ("Position"=w365:i32)  [unwired: 2 in]
        n181 = Number To Decimal String(number=w363) -> (decimal integer string=w373:string)  [unwired: 1 in]
        n182 = call "gsp_silvermax_writeregister.vi"("error in (no error)"=w362, "Register Value"=w365, "Motor #"=w370, "Register# (0)"=u8 25) -> ("error out"=w378:errorcluster, "Motor # dup"=w376:u8)  [unwired: 2 in]
        n183 = Build Array(w373) -> (w372:string[])
        n184 = call "gsp_silvermax_commandreponse.vi"("error in (no error)"=w378, "Parameters (none)"=w372, "Motor #"=w376, "Command"=T8."LRP (156)") -> ("error out"=w375:errorcluster)  [unwired: 3 out]
        n185 = case shown="No Error" w375 {
          selector: w375 -> [w381 w382]
          tunnel: [w381 w382] -> w374
          frame No Error {
            n186 = global write "GSP_Wavelength_Global.vi" "CS State"(MotorStates."Moving" ("Mode")) -> ()
          }
          frame Error {
          }
        }
      }
      frame "CAMERA_FLEX_MOVE_START" {
        w390 = 0.0  # Degrees
        n187 = Unflatten From String(type=w390, binary string=w391) -> (value=w383:dbl)  [unwired: 3 in, 2 out]
        n188 = global write "GSP_Wavelength_Global.vi" "Camera Flex Target"(w383) -> ()
        n189 = Unbundle By Name(w386) -> ("CS - Ext Move Mem Address"=w385:i32)
        n190 = global read "GSP_Wavelength_Global.vi" "CS - Degrees at Home"() -> (w388:dbl)
        n191 = global read "GSP_Wavelength_Global.vi" "CS - Ticks per Degree"() -> (w389:dbl)
        n192 = call "degreestopos.vi"("Degrees @ Home (15.00)"=w388, "Ticks per degree (28571.43)"=w389, "Degrees"=w383) -> ("Position"=w387:i32)  [unwired: 2 in]
        n193 = Number To Decimal String(number=w385) -> (decimal integer string=w395:string)  [unwired: 1 in]
        n194 = call "gsp_silvermax_writeregister.vi"("error in (no error)"=w384, "Register Value"=w387, "Motor #"=w392, "Register# (0)"=u8 25) -> ("error out"=w400:errorcluster, "Motor # dup"=w398:u8)  [unwired: 2 in]
        n195 = Build Array(w395) -> (w394:string[])
        n196 = call "gsp_silvermax_commandreponse.vi"("error in (no error)"=w400, "Parameters (none)"=w394, "Motor #"=w398, "Command"=T8."LRP (156)") -> ("error out"=w397:errorcluster)  [unwired: 3 out]
        n197 = case shown="No Error" w397 {
          selector: w397 -> [w403 w404]
          tunnel: [w403 w404] -> w396
          frame No Error {
            n198 = global write "GSP_Wavelength_Global.vi" "CS State"(MotorStates."Moving" ("Mode")) -> ()
          }
          frame Error {
          }
        }
      }
      frame "GRATING_EXT_MOVE_START" {
        w413 = 0.0  # Degrees
        n199 = Unflatten From String(type=w413, binary string=w414) -> (value=w405:dbl)  [unwired: 3 in, 2 out]
        n200 = global write "GSP_Wavelength_Global.vi" "Grating Target"(w405) -> ()
        n201 = local write "GS Target"(w405) -> ()
        n202 = Unbundle By Name(w408) -> ("GS - Move Mem Address"=w407:i32)
        n203 = global read "GSP_Wavelength_Global.vi" "GS - Ticks/Degree"() -> (w412:dbl)
        n204 = global read "GSP_Wavelength_Global.vi" "GS - Degrees at Home"() -> (w411:dbl)
        n205 = call "degreestopos.vi"("Degrees @ Home (15.00)"=w411, "Ticks per degree (28571.43)"=w412, "Degrees"=w405) -> ("Position"=w410:i32)  [unwired: 2 in]
        n206 = Number To Decimal String(number=w407) -> (decimal integer string=w417:string)  [unwired: 1 in]
        n207 = call "gsp_silvermax_writeregister.vi"("error in (no error)"=w406, "Register Value"=w410, "Motor #"=w409, "Register# (0)"=u8 25) -> ("error out"=w422:errorcluster, "Motor # dup"=w420:u8)  [unwired: 2 in]
        n208 = Build Array(w417) -> (w416:string[])
        n209 = call "gsp_silvermax_commandreponse.vi"("error in (no error)"=w422, "Parameters (none)"=w416, "Motor #"=w420, "Command"=T8."LRP (156)") -> ("error out"=w419:errorcluster)  [unwired: 3 out]
        n210 = case shown="No Error" w419 {
          selector: w419 -> [w425 w426]
          tunnel: [w425 w426] -> w418
          frame No Error {
            n211 = global write "GSP_Wavelength_Global.vi" "GS State"(MotorStates."Moving" ("Mode")) -> ()
          }
          frame Error {
          }
        }
      }
      frame "DUAL_MOVE_START" {
        n212 = Unflatten From String(type=T6 {"Camera Angle"=0.0, "Grating  Angle"=0.0, "Move type"=0} ("Wavelength Parameters"), binary string=w452) -> (value=w450:T6)  [unwired: 3 in, 2 out]
        n213 = Unbundle By Name(w450) -> ("Camera Angle"=w428:dbl, "Grating  Angle"=w427:dbl)
        n214 = global write "GSP_Wavelength_Global.vi" "Camera Target"(w428) -> ()
        n215 = local write "CS Target"(w428) -> ()
        n216 = Unbundle By Name(w448) -> ("CS - Int Move Mem Address"=w447:i32, "GS - Move Mem Address"=w439:i32)
        n217 = global write "GSP_Wavelength_Global.vi" "Grating Target"(w427) -> ()
        n218 = local write "GS Target"(w427) -> ()
        n219 = global read "GSP_Wavelength_Global.vi" "CS - Degrees at Home"() -> (w454:dbl)
        n220 = Number To Decimal String(number=w447) -> (decimal integer string=w458:string)  [unwired: 1 in]
        n221 = call "degreestopos.vi"("Degrees @ Home (15.00)"=w454, "Ticks per degree (28571.43)"=1960.0, "Degrees"=w428) -> ("Position"=w456:i32)  [unwired: 2 in]
        n222 = Build Array(w458) -> (w457:string[])
        n223 = call "gsp_silvermax_writeregister.vi"("error in (no error)"=w429, "Register Value"=w456, "Motor #"=w449, "Register# (0)"=u8 25) -> ("error out"=w459:errorcluster, "Motor # dup"=w431:u8)  [unwired: 2 in]
        n224 = call "gsp_silvermax_commandreponse.vi"("error in (no error)"=w459, "Parameters (none)"=w457, "Motor #"=w431, "Command"=T8."LRP (156)") -> ("error out"=w446:errorcluster)  [unwired: 3 out]
        n225 = global read "GSP_Wavelength_Global.vi" "GS - Ticks/Degree"() -> (w433:dbl)
        n226 = case shown="No Error" w446 {
          selector: w446 -> [w464 w466]
          tunnel: [w464 w466] -> w437
          frame No Error {
            n227 = global write "GSP_Wavelength_Global.vi" "CS State"(MotorStates."Moving" ("Mode")) -> ()
          }
          frame Error {
          }
        }
        n228 = global read "GSP_Wavelength_Global.vi" "GS - Degrees at Home"() -> (w436:dbl)
        n229 = call "degreestopos.vi"("Degrees @ Home (15.00)"=w436, "Ticks per degree (28571.43)"=w433, "Degrees"=w427) -> ("Position"=w432:i32)  [unwired: 2 in]
        n230 = Number To Decimal String(number=w439) -> (decimal integer string=w443:string)  [unwired: 1 in]
        n231 = call "gsp_silvermax_writeregister.vi"("error in (no error)"=w437, "Register Value"=w432, "Motor #"=w438, "Register# (0)"=u8 25) -> ("error out"=w444:errorcluster, "Motor # dup"=w430:u8)  [unwired: 2 in]
        n232 = Build Array(w443) -> (w442:string[])
        n233 = call "gsp_silvermax_commandreponse.vi"("error in (no error)"=w444, "Parameters (none)"=w442, "Motor #"=w430, "Command"=T8."LRP (156)") -> ("error out"=w440:errorcluster)  [unwired: 3 out]
        n234 = case shown="No Error" w440 {
          selector: w440 -> [w462 w463]
          tunnel: [w462 w463] -> w434
          frame No Error {
            n235 = global write "GSP_Wavelength_Global.vi" "GS State"(MotorStates."Moving" ("Mode")) -> ()
          }
          frame Error {
          }
        }
      }
      frame "SHUTDOWN" {
        n236 = global read "GSP_Wavelength_Global.vi" "Wavelength Thread State"() -> (w467:T10)
        n237 = case shown="\"Error\"" w467 {
          tunnel: w472 -> [w486 w500 w504 w508]
          tunnel: [w485 w499 w504 w508] -> w468
          tunnel: w471 -> [_ _ w503 w507]
          tunnel: [w484 w498 w502 w506] -> w470
          tunnel: w469 -> [w484 w498 _ _]
          frame "Waiting", Default {
            w476 = T7 0 items=["Both", "Grating Only", "Camera Only"] ("Move type")
            n238 = global read "GSP_Wavelength_Global.vi" "Camera Angle"() -> (w477:dbl)
            n239 = global read "GSP_Wavelength_Global.vi" "Grating Angle"() -> (w482:dbl)
            n240 = global read "GSP_Wavelength_Global.vi" "CS - Degrees at Home"() -> (w480:dbl)
            n241 = global read "GSP_Wavelength_Global.vi" "GS - Degrees at Home"() -> (w481:dbl)
            n242 = call "GSP_Wavelength_GenerateScript.vi"("Current Grating"=w482, "Current Camera"=w477, "Target Grating"=w481, "Target Camera"=w480, "Move type"=w476) -> ("Script"=w479:cluster{string, string}[])  [unwired: 1 out]
            n243 = Build Array (concatenate)(cluster{string, string} {"START_SCRIPT", ""}, w479, cluster{string, string} {"END_SCRIPT", ""}, cluster{string, string} {"FINAL_SHUTDOWN", ""}) -> (w478:cluster{string, string}[])
            n244 = call "Build_Script.vi"("Commands"=w478) -> ("script out"=w483:T3)  [unwired: 4 in]
            n245 = Insert Into Array(array=w486, new element=w483) -> (w485:T2)  [unwired: 1 in]
          }
          frame "Scripting" {
            w490 = T7 0 items=["Both", "Grating Only", "Camera Only"] ("Move type")
            n246 = global read "GSP_Wavelength_Global.vi" "Camera Angle"() -> (w491:dbl)
            n247 = global read "GSP_Wavelength_Global.vi" "Grating Angle"() -> (w496:dbl)
            n248 = global read "GSP_Wavelength_Global.vi" "CS - Degrees at Home"() -> (w494:dbl)
            n249 = global read "GSP_Wavelength_Global.vi" "GS - Degrees at Home"() -> (w495:dbl)
            n250 = call "GSP_Wavelength_GenerateScript.vi"("Current Grating"=w496, "Current Camera"=w491, "Target Grating"=w495, "Target Camera"=w494, "Move type"=w490) -> ("Script"=w493:cluster{string, string}[])  [unwired: 1 out]
            n251 = Build Array (concatenate)(cluster{string, string} {"START_SCRIPT", ""}, w493, cluster{string, string} {"END_SCRIPT", ""}, cluster{string, string} {"FINAL_SHUTDOWN", ""}) -> (w492:cluster{string, string}[])
            n252 = call "Build_Script.vi"("Commands"=w492) -> ("script out"=w497:T3)  [unwired: 4 in]
            n253 = Insert Into Array(array=w500, new element=w497) -> (w499:T2)  [unwired: 1 in]
          }
          frame "Uninitialized" {
            n254 = Enqueue Element At Opposite End(queue=w503, element=T4 {"Command"="FINAL_SHUTDOWN", "Parameter"=""}) -> (error out=w502:errorcluster)  [unwired: 2 in, 2 out]
          }
          frame "Error" {
            n255 = Enqueue Element At Opposite End(queue=w507, element=T4 {"Command"="FINAL_SHUTDOWN", "Parameter"=""}) -> (error out=w506:errorcluster)  [unwired: 2 in, 2 out]
          }
        }
      }
      frame "FINAL_SHUTDOWN" {
        n256 = Release Queue(queue=w514, error in (no error)=w515) -> (error out=w511:errorcluster)  [unwired: 1 in, 2 out]
        n257 = global write "GSP_Wavelength_Global.vi" "Wavelength Thread State"(ThreadStates."Uninitialized" ("Thread state")) -> ()
        n258 = property on="Select Mode:" class="Ring (strict)"(error in=w511, "Disabled"=u8 2) -> (error out=w510:errorcluster)  [unwired: 1 in, 1 out]
        n259 = stacked-sequence {
          tunnel: w510 -> [_]
          frame #0 {
            n260 = global write "GSP_Wavelength_Global.vi" "WL Online"(FALSE ("CS Online")) -> ()
          }
        }
      }
      frame "HOME" {
        w517 = MotorStates."Ready" ("Camera Mode")
        n261 = call "Build_Script.vi"("Commands"=cluster{"Command":string, "Parameters":string}[] [{"Command"="START_SCRIPT", "Parameters"=""}, {"Command"="HOME_START", "Parameters"=""}, {"Command"="END_SCRIPT", "Parameters"=""}]) -> ("script out"=w519:T3)  [unwired: 4 in]
        n262 = Insert Into Array(array=w521, new element=w519) -> (w520:T2)  [unwired: 1 in]
        n263 = global write "GSP_Wavelength_Global.vi" "GS State"(w517) -> ()
        n264 = global write "GSP_Wavelength_Global.vi" "CS State"(w517) -> ()
      }
      frame "HOME_START" {
        n265 = Unbundle By Name(w526) -> ("GS - Home Mem Address"=w525:i32, "CS - Home Mem Address"=w524:i32)
        n266 = Number To Decimal String(number=w524) -> (decimal integer string=w536:string)  [unwired: 1 in]
        n267 = Build Array(w536) -> (w535:string[])
        n268 = Number To Decimal String(number=w525) -> (decimal integer string=w532:string)  [unwired: 1 in]
        n269 = call "gsp_silvermax_commandreponse.vi"("error in (no error)"=w523, "Parameters (none)"=w535, "Motor #"=w528, "Command"=T8."LRP (156)") -> ("error out"=w530:errorcluster)  [unwired: 3 out]
        n270 = Build Array(w532) -> (w531:string[])
        n271 = call "gsp_silvermax_commandreponse.vi"("error in (no error)"=w530, "Parameters (none)"=w531, "Motor #"=w527, "Command"=T8."LRP (156)") -> ("error out"=w529:errorcluster)  [unwired: 3 out]
        n272 = case shown="No Error" w529 {
          selector: w529 -> [w542 w543]
          tunnel: [w542 w543] -> w537
          frame No Error {
            w541 = MotorStates."Moving" ("Mode")
            n273 = global read "GSP_Wavelength_Global.vi" "CS - Degrees at Home"() -> (w540:dbl)
            n274 = global write "GSP_Wavelength_Global.vi" "Camera Target"(w540) -> ()
            n275 = local write "CS Target"(w540) -> ()
            n276 = global read "GSP_Wavelength_Global.vi" "GS - Degrees at Home"() -> (w539:dbl)
            n277 = global write "GSP_Wavelength_Global.vi" "Grating Target"(w539) -> ()
            n278 = local write "GS Target"(w539) -> ()
            n279 = global write "GSP_Wavelength_Global.vi" "GS State"(w541) -> ()
            n280 = global write "GSP_Wavelength_Global.vi" "CS State"(w541) -> ()
          }
          frame Error {
          }
        }
      }
      frame "ERROR" {
        n281 = local read "Last Error"() -> (w548:errorcluster)
        n282 = Unbundle By Name(w548) -> ("code"=w553:i32)
        n283 = Bundle By Name(cluster=T12 {"error in (no error)"={"status"=FALSE, "code"=0, "source"=""}, "Source"="", "Comment "=""} ("Log"), "error in (no error)"=w548, "Source"="Wavlength Manager") -> (w549:T12)
        n284 = call "GSP_Logger_Handler.vi"("Log"=w549, "Actions"=T11."Log") -> ()  [unwired: 5 in, 1 out]
        n285 = case shown="5003, 5006" w553 {
          tunnel: w548 -> [_ _ _]
          tunnel: [errorcluster {"status"=FALSE, "code"=0, "source"=""} ("Last Error") errorcluster {"status"=FALSE, "code"=0, "source"=""} ("Last Error") errorcluster {"status"=FALSE, "code"=0, "source"=""} ("Last Error")] -> w547
          tunnel: w545 -> [_ w562 w564]
          tunnel: [T2 [] ("Operations") w562 w564] -> w544
          frame 0, Default {
            w559 = MotorStates."Error" ("Mode")
            n286 = global write "GSP_Wavelength_Global.vi" "GS State"(w559) -> ()
            n287 = global write "GSP_Wavelength_Global.vi" "CS State"(w559) -> ()
            n288 = property on="Select Mode:" class="Ring (strict)"("Disabled"=u8 2) -> ()  [unwired: 2 in, 2 out]
            n289 = global write "GSP_Wavelength_Global.vi" "Wavelength Thread State"(ThreadStates."Error" ("Thread state")) -> ()
          }
          frame 5003, 5006 {
          }
          frame 5013 {
          }
        }
        n290 = case shown="Error" w547 {
          tunnel: w552 -> [_ w555]
          frame No Error {
          }
          frame Error {
            n291 = Enqueue Element At Opposite End(queue=w555, element=T4 {"Command"="FINAL_SHUTDOWN", "Parameter"=""}) -> ()  [unwired: 2 in, 3 out]
          }
        }
      }
    }
    n292 = Equal?(x=w23, y="FINAL_SHUTDOWN") -> (x = y?=w22:bool)
    n293 = case shown="Error" w30 {
      selector: w30 -> [_ w38]
      tunnel: w29 -> [_ w39]
      tunnel: w23 -> [_ w35]
      frame No Error {
      }
      frame Error {
        n294 = Bundle By Name(cluster=T4 {"Command"="", "Parameter"=""} ("Command"), "Command"="ERROR" ("element"), "Parameter"=w35) -> (w36:T4)
        n295 = Enqueue Element At Opposite End(queue=w39, element=w36) -> ()  [unwired: 2 in, 3 out]
        "Last Error" <- w38
      }
    }
  }
  n296 = control-ref of="Select Mode:"() -> (w1:refnum<vi>)
  n297 = global write "GSP_Wavelength_Global.vi" "WAVMODE REF"(w1) -> ()
